vi "Default Settings.vi"(6 "Assembly Type":string, 8 "error in (no error)":errorcluster, 11 "Pick and Place in":refnum<class "Pick and Place.lvclass">) -> (0 "error out":errorcluster, 3 "Pick and Place out":refnum<class "Pick and Place.lvclass">)   [LabVIEW 2021, in "Pick and Place.lvclass"]
uses:
  Pick and Place.lvclass
panel:
  # "This Routine does not Accept Settings"
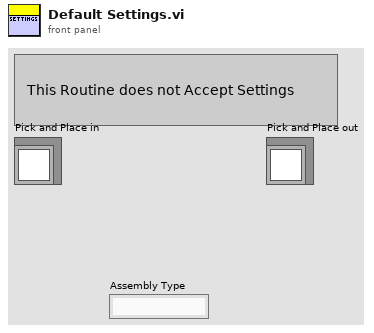
[diagram p1: front panel]
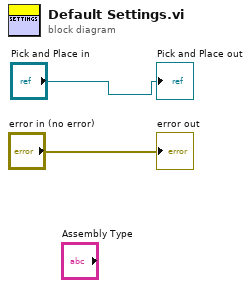
[diagram p0: block diagram]
diagram:
  "error out" <- "error in (no error)"
  "Pick and Place out" <- "Pick and Place in"
